vi "OxITC503_Read0167.vi"(0 "VISA session 2":refnum<visa-resource-name>, 11 "error in":errorcluster) -> (4 "Temp":dbl format="%.2f", 6 "SetPoint":dbl format="%.2f", 8 "Heater\nOutput":dbl format="%.2f", 10 "GasFlow":dbl format="%.2f", 14 "VISA session":refnum<visa-resource-name>, 15 "error out (no error)":errorcluster)   [LabVIEW 2014]
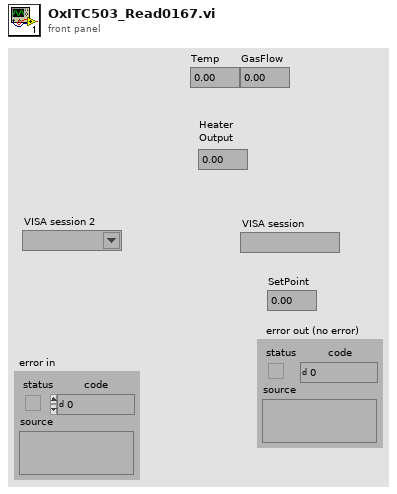
[diagram p1: front panel]
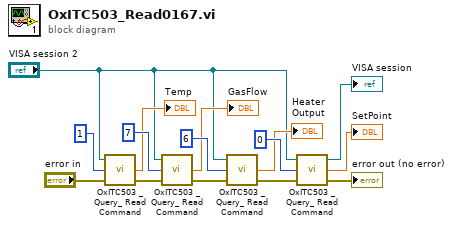
[diagram p0: block diagram]
diagram:
  n1 = call "OxITC503 _Query_ Read Command.vi"("error in"="error in", "Read Item"=1, "VISA session"="VISA session 2") -> ("error out (no error)"=w13:errorcluster, "Output of Read"=→"Temp":dbl)  [unwired: 1 out]
  n2 = call "OxITC503 _Query_ Read Command.vi"("error in"=w13, "Read Item"=7, "VISA session"="VISA session 2") -> ("error out (no error)"=w11:errorcluster, "Output of Read"=→"GasFlow":dbl)  [unwired: 1 out]
  n3 = call "OxITC503 _Query_ Read Command.vi"("error in"=w11, "Read Item"=6, "VISA session"="VISA session 2") -> ("error out (no error)"=w9:errorcluster, "Output of Read"=→"Heater\nOutput":dbl)  [unwired: 1 out]
  n4 = call "OxITC503 _Query_ Read Command.vi"("error in"=w9, "Read Item"=0, "VISA session"="VISA session 2") -> ("error out (no error)"=→"error out (no error)":errorcluster, "Output of Read"=→"SetPoint":dbl, "VISA session"=→"VISA session":refnum<visa-resource-name>)
